vi "Search Cave Type.vi"(10 "Type":T2, 11 "Array":T1[](array[typedef])) -> (2 "Found?":bool, 3 "Cave":T1)   [LabVIEW 2019, in "Day 12.lvlib"]
uses:
  Day 12.lvlib
  Controls/Cave Type.ctl
  Controls/Cave.ctl
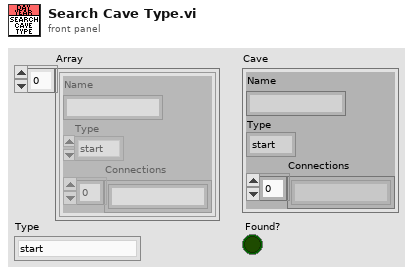
[diagram p1: front panel]
types:
  T1 = typedef "Day 12.lvlib/Cave.ctl" = cluster{"Name":string, "Type":T2, "Connections":string[]}
  T2 = typedef "Day 12.lvlib/Cave Type.ctl" = enum16{"start", "end", "small", "big"}
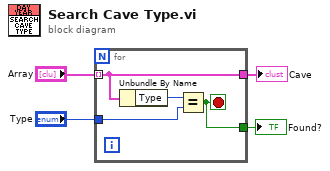
[diagram p0: block diagram]
diagram:
  n1 = for {
    tunnel: "Array" -> [w7] mode=indexing
    tunnel: [w7] -> w1
    tunnel: "Type" -> [w6]
    tunnel: [w5] -> w2
    stop <- w5 stop-if-true
    n2 = Unbundle By Name(w7) -> ("Type"=w8:T2)
    n3 = Equal?(x=w8, y=w6) -> (x = y?=w5:bool)
  }
  "Found?" <- w2
  "Cave" <- w1
